vi "RS232 485发送接收.vi"() -> ()   [LabVIEW 2010]
uses:
  <vilib>/Instr/_visa.llb/VISA Configure Serial Port (Instr).vi
panel:
  out "接收数据_3":string
  out "成功_3？":bool caption="成功？"
  in  "发送数据_3":string
  out "接收数据_2":string
  out "成功_2？":bool caption="成功？"
  in  "发送数据_2":string
  in  "btn_关闭":bool
  in  "btn_开始测试":bool
  out "接收数据_1":string
  out "成功_1？":bool caption="成功？"
  in  "发送数据_1":string
  # "RS232测试界面"
  # "1#发送字符"
  # "2#发送字符"
  # "1#接收字符"
  # "2#接收字符"
  # "1#测试结果"
  # "2#测试结果"
  # "RS485测试界面"
  # "1#发送字符"
  # "1#接收字符"
  # "1#测试结果"
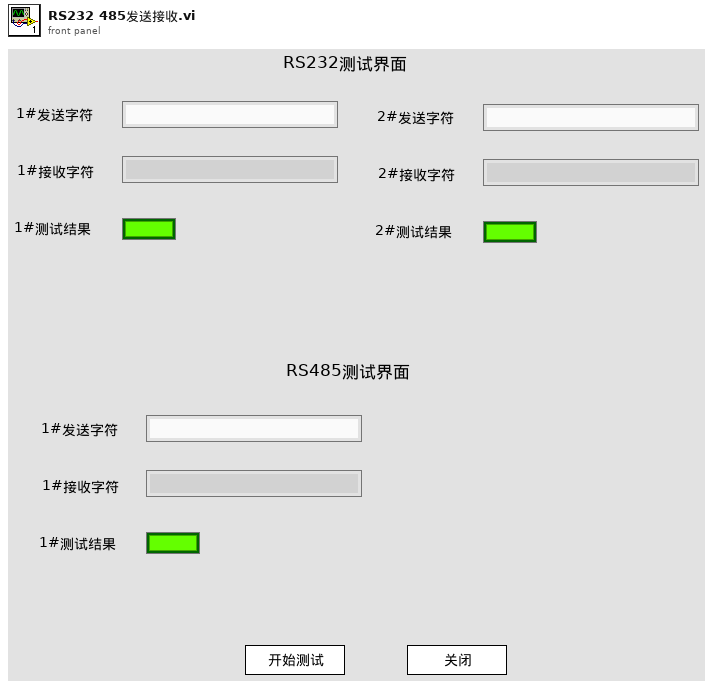
[diagram p1: front panel]
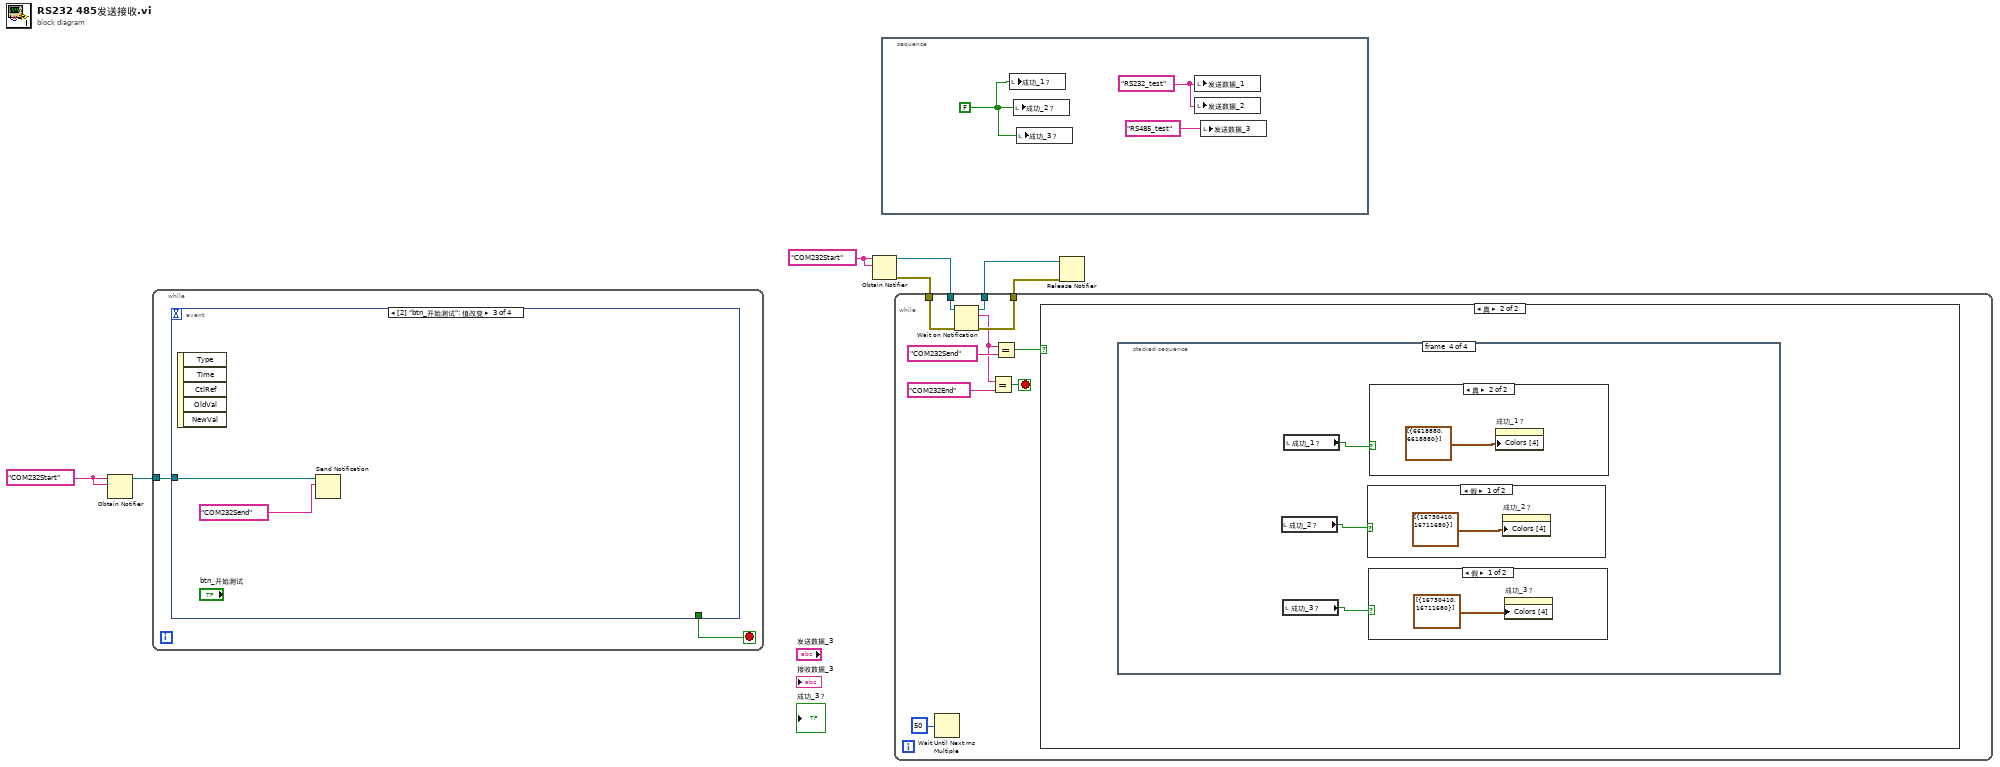
[diagram p0: block diagram]
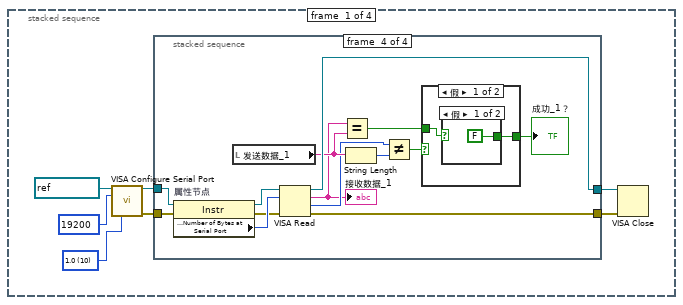
[diagram p3: hidden frame]
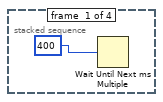
[diagram p4: hidden frame]
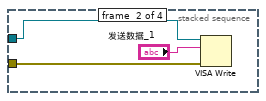
[diagram p5: hidden frame]
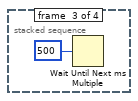
[diagram p6: hidden frame]
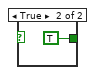
[diagram p7: hidden frame]
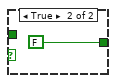
[diagram p8: hidden frame]
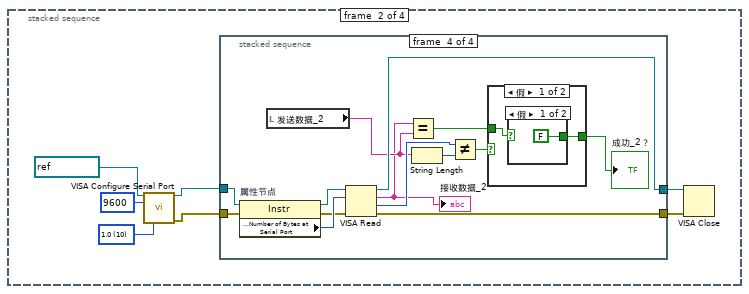
[diagram p9: hidden frame]
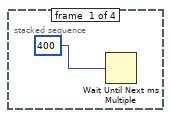
[diagram p10: hidden frame]
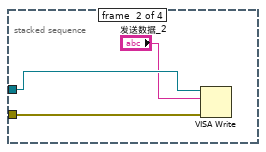
[diagram p11: hidden frame]
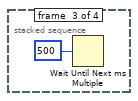
[diagram p12: hidden frame]
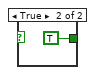
[diagram p13: hidden frame]
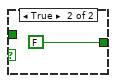
[diagram p14: hidden frame]
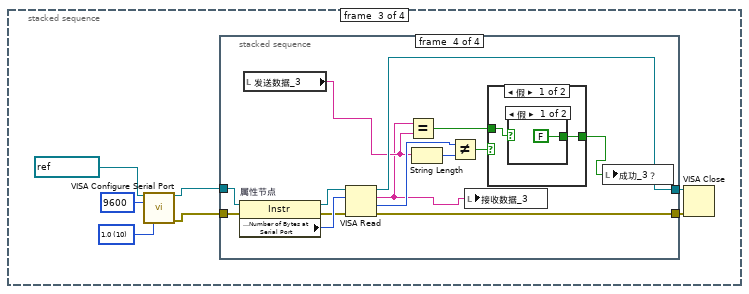
[diagram p15: hidden frame]
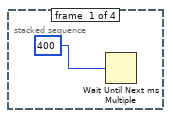
[diagram p16: hidden frame]
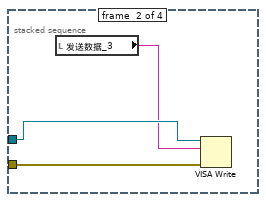
[diagram p17: hidden frame]
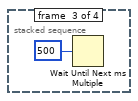
[diagram p18: hidden frame]
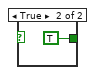
[diagram p19: hidden frame]
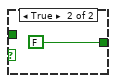
[diagram p20: hidden frame]
diagram:
  w2 = "COM232Start" ("名称（未命名）")
  w7 = "COM232Start" ("名称（未命名）")
  n1 = Obtain Notifier(name (unnamed)=w2, notification data type=w2) -> (notifier out=w1:refnum<notifier>)  [unwired: 2 in, 2 out]
  n2 = while {
    tunnel: w1 -> [w8]
    stop <- w9 stop-if-true
    n3 = event shown="[2] \"btn_开始测试\": 值改变" {
      selector: _ -> [_ _ _ _]
      dyn-events: _ -> [_ _ _ _]
      timeout: _ -> [_ _ _ _]
      tunnel: [_ TRUE _ TRUE] -> w9
      tunnel: w8 -> [_ w11 w13 w15]
      event Timeout {
        n4 = event-data() -> ()  [unwired: 1 in, 2 out]
      }
      event Panel Close {
        n5 = event-data() -> ()  [unwired: 1 in, 3 out]
        n6 = Send Notification(notification="COM232End" ("通知"), notifier=w11) -> ()  [unwired: 1 in, 2 out]
      }
      event "btn_开始测试": Value Change {
        n7 = event-data() -> ()  [unwired: 1 in, 5 out]
        n8 = Send Notification(notification="COM232Send" ("通知"), notifier=w13) -> ()  [unwired: 1 in, 2 out]
      }
      event "btn_关闭": Value Change {
        n9 = event-data() -> ()  [unwired: 1 in, 5 out]
        n10 = Send Notification(notification="COM232End" ("通知"), notifier=w15) -> ()  [unwired: 1 in, 2 out]
      }
    }
  }
  n11 = Obtain Notifier(name (unnamed)=w7, notification data type=w7) -> (notifier out=w6:refnum<notifier>, error out=w5:errorcluster)  [unwired: 2 in, 1 out]
  n12 = stacked-sequence {
    frame #0 {
      w18 = FALSE
      w20 = "RS232_test" ("发送数据_1")
      n13 = local write "成功_1？"(w18) -> ()
      n14 = local write "成功_2？"(w18) -> ()
      n15 = local write "成功_3？"(w18) -> ()
      n16 = local write "发送数据_1"(w20) -> ()
      n17 = local write "发送数据_2"(w20) -> ()
      n18 = local write "发送数据_3"("RS485_test" ("发送数据_1")) -> ()
    }
  }
  n19 = while {
    tunnel: w6 -> [w30]
    tunnel: w5 -> [w29]
    tunnel: [w28] -> w4
    tunnel: [w27] -> w3
    stop <- w22 stop-if-true
    n20 = Wait Until Next ms Multiple(millisecond multiple=u32 50 ("毫秒倍数")) -> ()  [unwired: 1 out]
    n21 = Wait on Notification(notifier=w30, error in (no error)=w29) -> (notifier out=w28:refnum<notifier>, notification=w24:string, error out=w27:errorcluster)  [unwired: 2 in, 1 out]
    n22 = Equal?(x=w24, y="COM232End" ("通知")) -> (x = y?=w22:bool)
    n23 = Equal?(x=w24, y="COM232Send" ("通知")) -> (x = y?=w25:bool)
    n24 = case shown="真" w25 {
      frame False {
      }
      frame True {
        n25 = stacked-sequence {
          frame #0 {
            w35 = u16 10 items=["1.0"=10, "1.5"=15, "2.0"=20] ("stop bits (10: 1 bit)")
            n26 = call-poly "VISA Configure Serial Port"("VISA resource name"=refnum<visa-resource-name> "COM1" ("R232端口"), "baud rate (9600)"=u32 19200, "stop bits (10: 1 bit)"=w35) -> ("VISA resource name out"=w34:refnum<visa-resource-name>, "error out"=w33:errorcluster)  [unwired: 11 in]
            n27 = stacked-sequence {
              tunnel: w34 -> [_ w41 _ w54]
              tunnel: w33 -> [_ w40 _ w53]
              tunnel: [_ _ _ w56] -> w32
              tunnel: [_ _ _ w55] -> w31
              frame #0 {
                n28 = Wait Until Next ms Multiple(millisecond multiple=u32 400 ("毫秒倍数")) -> ()  [unwired: 1 out]
              }
              frame #1 {
                n29 = VISA Write(VISA resource name=w41, write buffer="发送数据_1", error in (no error)=w40) -> ()  [unwired: 3 out]
              }
              frame #2 {
                n30 = Wait Until Next ms Multiple(millisecond multiple=u32 500 ("毫秒倍数")) -> ()  [unwired: 1 out]
              }
              frame #3 {
                n31 = property on="属性节点" class="Instr"(reference=w54, error in=w53) -> (reference out=w50:refnum<visa-resource-name>, error out=w48:errorcluster, "Serial Settings:Number of Bytes at Serial Port"=w49:u32)
                n32 = local read "发送数据_1"() -> (w47:string)
                n33 = VISA Read(VISA resource name=w50, byte count=w49, error in (no error)=w48) -> (VISA resource name out=w56:refnum<visa-resource-name>, read buffer=w43:string, return count=w46:u32, error out=w55:errorcluster)
                "接收数据_1" <- w43
                n34 = Equal?(x=w43, y=w47) -> (x = y?=w52:bool)
                n35 = String Length(string=w47) -> (length=w45:i32)
                n36 = Not Equal?(x=w46, y=w45) -> (x != y?=w44:bool)
                n37 = case shown="假" w44 {
                  tunnel: w52 -> [w58 _]
                  tunnel: [w57 FALSE] -> w51
                  frame False {
                    n38 = case shown="假" w58 {
                      tunnel: [FALSE TRUE] -> w57
                      frame False {
                      }
                      frame True {
                      }
                    }
                  }
                  frame True {
                  }
                }
                "成功_1？" <- w51
              }
            }
            n39 = VISA Close(VISA resource name=w32, error in (no error)=w31) -> ()  [unwired: 1 out]
          }
          frame #1 {
            w66 = u16 10 items=["1.0"=10, "1.5"=15, "2.0"=20] ("stop bits (10: 1 bit)")
            n40 = call-poly "VISA Configure Serial Port"("VISA resource name"=refnum<visa-resource-name> "COM3" ("R232端口"), "baud rate (9600)"=u32 9600, "stop bits (10: 1 bit)"=w66) -> ("VISA resource name out"=w63:refnum<visa-resource-name>, "error out"=w62:errorcluster)  [unwired: 11 in]
            n41 = stacked-sequence {
              tunnel: w63 -> [_ w72 _ w85]
              tunnel: w62 -> [_ w71 _ w84]
              tunnel: [_ _ _ w87] -> w68
              tunnel: [_ _ _ w86] -> w67
              frame #0 {
                n42 = Wait Until Next ms Multiple(millisecond multiple=u32 400 ("毫秒倍数")) -> ()  [unwired: 1 out]
              }
              frame #1 {
                n43 = VISA Write(VISA resource name=w72, write buffer="发送数据_2", error in (no error)=w71) -> ()  [unwired: 3 out]
              }
              frame #2 {
                n44 = Wait Until Next ms Multiple(millisecond multiple=u32 500 ("毫秒倍数")) -> ()  [unwired: 1 out]
              }
              frame #3 {
                n45 = property on="属性节点" class="Instr"(reference=w85, error in=w84) -> (reference out=w82:refnum<visa-resource-name>, error out=w80:errorcluster, "Serial Settings:Number of Bytes at Serial Port"=w81:u32)
                n46 = local read "发送数据_2"() -> (w76:string)
                n47 = VISA Read(VISA resource name=w82, byte count=w81, error in (no error)=w80) -> (VISA resource name out=w87:refnum<visa-resource-name>, read buffer=w75:string, return count=w79:u32, error out=w86:errorcluster)
                "接收数据_2" <- w75
                n48 = Equal?(x=w75, y=w76) -> (x = y?=w83:bool)
                n49 = String Length(string=w76) -> (length=w78:i32)
                n50 = Not Equal?(x=w79, y=w78) -> (x != y?=w77:bool)
                n51 = case shown="假" w77 {
                  tunnel: w83 -> [w89 _]
                  tunnel: [w88 FALSE] -> w74
                  frame False {
                    n52 = case shown="假" w89 {
                      tunnel: [FALSE TRUE] -> w88
                      frame False {
                      }
                      frame True {
                      }
                    }
                  }
                  frame True {
                  }
                }
                "成功_2？" <- w74
              }
            }
            n53 = VISA Close(VISA resource name=w68, error in (no error)=w67) -> ()  [unwired: 1 out]
          }
          frame #2 {
            w97 = u16 10 items=["1.0"=10, "1.5"=15, "2.0"=20] ("stop bits (10: 1 bit)")
            n54 = call-poly "VISA Configure Serial Port"("VISA resource name"=refnum<visa-resource-name> "COM4" ("R232端口"), "baud rate (9600)"=u32 9600, "stop bits (10: 1 bit)"=w97) -> ("VISA resource name out"=w94:refnum<visa-resource-name>, "error out"=w93:errorcluster)  [unwired: 11 in]
            n55 = stacked-sequence {
              tunnel: w94 -> [_ w103 _ w116]
              tunnel: w93 -> [_ w102 _ w115]
              tunnel: [_ _ _ w118] -> w99
              tunnel: [_ _ _ w117] -> w98
              frame #0 {
                n56 = Wait Until Next ms Multiple(millisecond multiple=u32 400 ("毫秒倍数")) -> ()  [unwired: 1 out]
              }
              frame #1 {
                n57 = local read "发送数据_3"() -> (w101:string)
                n58 = VISA Write(VISA resource name=w103, write buffer=w101, error in (no error)=w102) -> ()  [unwired: 3 out]
              }
              frame #2 {
                n59 = Wait Until Next ms Multiple(millisecond multiple=u32 500 ("毫秒倍数")) -> ()  [unwired: 1 out]
              }
              frame #3 {
                n60 = property on="属性节点" class="Instr"(reference=w116, error in=w115) -> (reference out=w113:refnum<visa-resource-name>, error out=w111:errorcluster, "Serial Settings:Number of Bytes at Serial Port"=w112:u32)
                n61 = local read "发送数据_3"() -> (w107:string)
                n62 = VISA Read(VISA resource name=w113, byte count=w112, error in (no error)=w111) -> (VISA resource name out=w118:refnum<visa-resource-name>, read buffer=w106:string, return count=w110:u32, error out=w117:errorcluster)
                n63 = Equal?(x=w106, y=w107) -> (x = y?=w114:bool)
                n64 = String Length(string=w107) -> (length=w109:i32)
                n65 = Not Equal?(x=w110, y=w109) -> (x != y?=w108:bool)
                n66 = local write "接收数据_3"(w106) -> ()
                n67 = case shown="假" w108 {
                  tunnel: w114 -> [w120 _]
                  tunnel: [w119 FALSE] -> w105
                  frame False {
                    n68 = case shown="假" w120 {
                      tunnel: [FALSE TRUE] -> w119
                      frame False {
                      }
                      frame True {
                      }
                    }
                  }
                  frame True {
                  }
                }
                n69 = local write "成功_3？"(w105) -> ()
              }
            }
            n70 = VISA Close(VISA resource name=w99, error in (no error)=w98) -> ()  [unwired: 1 out]
          }
          frame #3 {
            n71 = local read "成功_2？"() -> (w125:bool)
            n72 = local read "成功_3？"() -> (w124:bool)
            n73 = local read "成功_1？"() -> (w126:bool)
            n74 = case shown="假" w125 {
              frame False {
                n75 = property on="成功_2？" class="Bool (严格)"("Colors [4]"=cluster{u32, u32}[] [{16730410, 16711680}]) -> ()  [unwired: 2 in, 2 out]
              }
              frame True {
                n76 = property on="成功_2？" class="Bool (严格)"("Colors [4]"=cluster{u32, u32}[] [{6618880, 6618880}]) -> ()  [unwired: 2 in, 2 out]
              }
            }
            n77 = case shown="假" w124 {
              frame False {
                n78 = property on="成功_3？" class="Bool (严格)"("Colors [4]"=cluster{u32, u32}[] [{16730410, 16711680}]) -> ()  [unwired: 2 in, 2 out]
              }
              frame True {
                n79 = property on="成功_3？" class="Bool (严格)"("Colors [4]"=cluster{u32, u32}[] [{6618880, 6618880}]) -> ()  [unwired: 2 in, 2 out]
              }
            }
            n80 = case shown="真" w126 {
              frame False {
                n81 = property on="成功_1？" class="Bool (严格)"("Colors [4]"=cluster{u32, u32}[] [{16730410, 16711680}]) -> ()  [unwired: 2 in, 2 out]
              }
              frame True {
                n82 = property on="成功_1？" class="Bool (严格)"("Colors [4]"=cluster{u32, u32}[] [{6618880, 6618880}]) -> ()  [unwired: 2 in, 2 out]
              }
            }
          }
        }
      }
    }
  }
  n83 = Release Notifier(notifier=w4, error in (no error)=w3) -> ()  [unwired: 1 in, 3 out]
